vi "Check Escala.vi"(8 "error in (no error)":errorcluster, 10 "Grandeza":string, 11 "Multimeter in":refnum<class "Multimeter.lvclass">) -> (0 "error out":errorcluster, 2 "Escala Correta?":bool, 3 "Multimeter out":refnum<class "Multimeter.lvclass">)   [LabVIEW 2015, in "Multimeter.lvclass"]
uses:
  Multimeter.lvclass
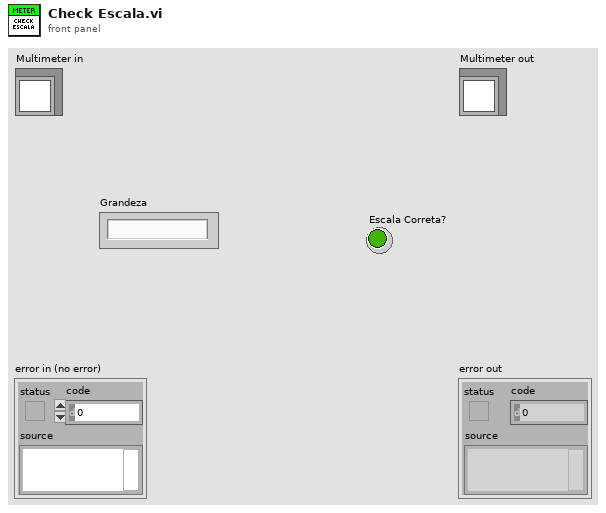
[diagram p1: front panel]
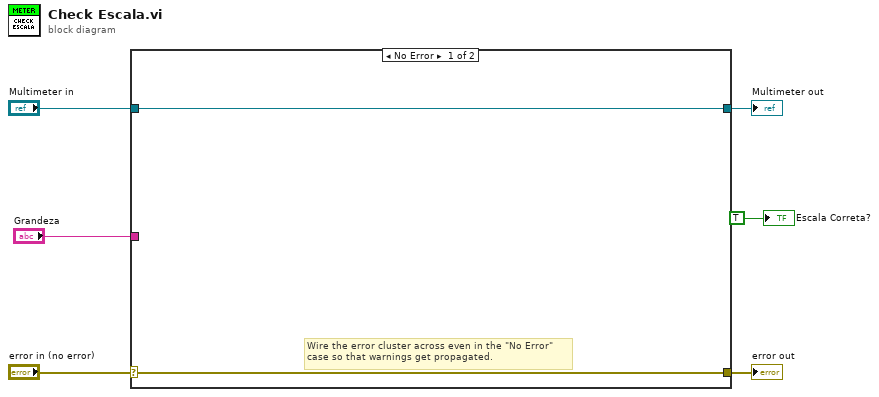
[diagram p0: block diagram]
diagram:
  n1 = case shown="No Error" "error in (no error)" {
    selector: "error in (no error)" -> [w7 w10]
    tunnel: [w7 w10] -> w5
    tunnel: [w8 w9] -> w3
    tunnel: "Multimeter in" -> [w8 w9]
    tunnel: "Grandeza" -> [_ _]
    frame No Error {
      # "Wire the error cluster across even in the \"No Error\"\ncase so that warnings get propagated."
    }
    frame Error {
    }
  }
  "error out" <- w5
  "Multimeter out" <- w3
  "Escala Correta?" <- TRUE
